vi "MW100 General ReBoot.vi"(8 "error in (no error)":errorcluster, 11 "VISA Refnum in":refnum<visa-resource-name>) -> (0 "error out":errorcluster, 3 "VISA Refnum out":refnum<visa-resource-name>)   [LabVIEW 2020]
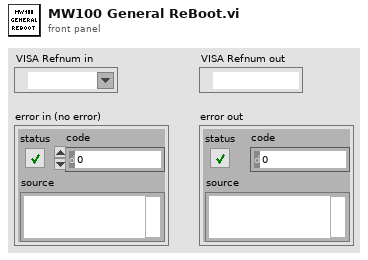
[diagram p1: front panel]
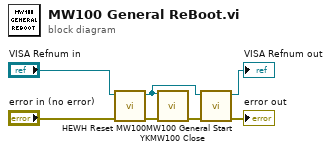
[diagram p0: block diagram]
diagram:
  n1 = call "HEWH Reset MW100.vi"("error in (no error)"="error in (no error)", "MW100 VISA In"="VISA Refnum in") -> ("error out"=w3:errorcluster, "MW100 VISA Out"=w6:refnum<visa-resource-name>)  [unwired: 8 in]
  n2 = call "YKMW100 Close.vi"("VISA session"=w6, "error in (no error)"=w3) -> ("error out"=w4:errorcluster)  [unwired: 13 in]
  n3 = call "MW100 General Start.vi"("error in (no error)"=w4, "MW100 Input"=w6) -> ("error out"=→"error out":errorcluster, "MW100 Output"=→"VISA Refnum out":refnum<visa-resource-name>)  [unwired: 8 in]
